vi "Inst_DS360.vi"(8 "error in":errorcluster, 10 "All Message Queues in":T1, 11 "AjustesPrevios in":refnum<class "AjustesPrevios.lvclass">) -> (0 "error out":errorcluster)   [LabVIEW 2019, in "AjustesPrevios.lvclass"]
uses:
  AjustesPrevios.lvclass
  QMH/Message Queue/All Message Queues.ctl
  QMH/Message Queue/Message Cluster.ctl
  AjustesPrevios.lvclass/AjustesPrevios.ctl
  <vilib>/Utility/error.llb/Error Cluster From Error Code.vi
  QMH/Message Queue/Enqueue Message (Single).vi
  <vilib>/ErrorRing/Error Ring.xnode
  QMH/Message Queue/Message Queue.lvlib
  Instrumento/DS360/DS360.lvclass
panel:
  out "All States":string[](array[string])
  out "Actual State":string
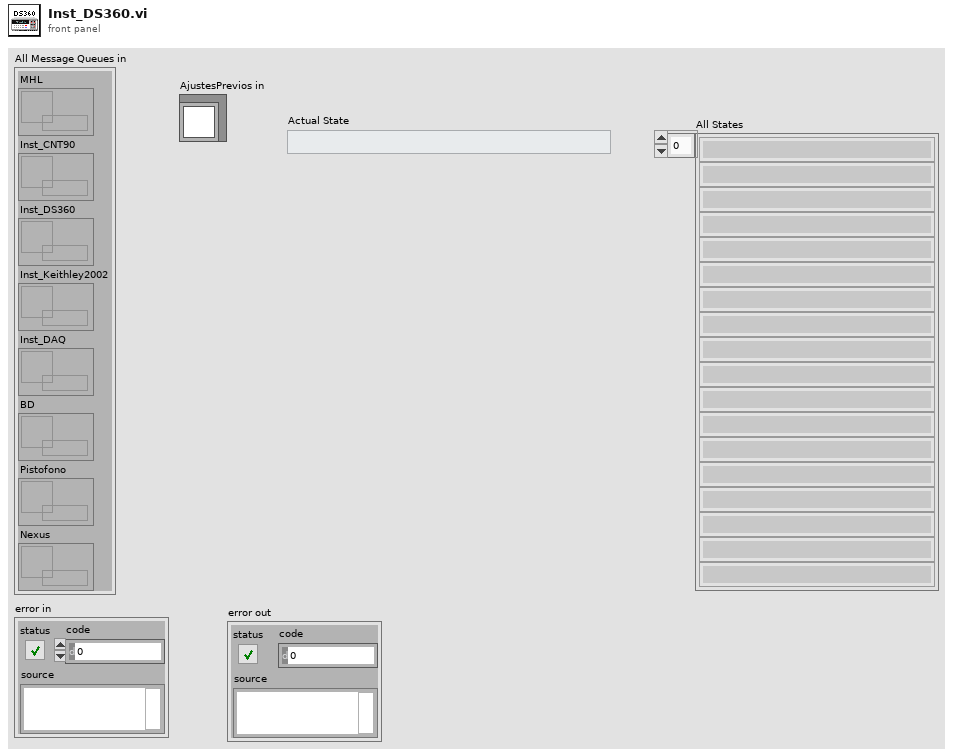
[diagram p1: front panel]
types:
  T1 = typedef "Message Queue.lvlib/All Message Queues.ctl" = cluster{"MHL":refnum<queue>, "Inst_CNT90":refnum<queue>, "Inst_DS360":refnum<queue>, "Inst_Keithley2002":refnum<queue>, "Inst_DAQ":refnum<queue>, "BD":refnum<queue>, "Pistofono":refnum<queue>, "Nexus":refnum<queue>}
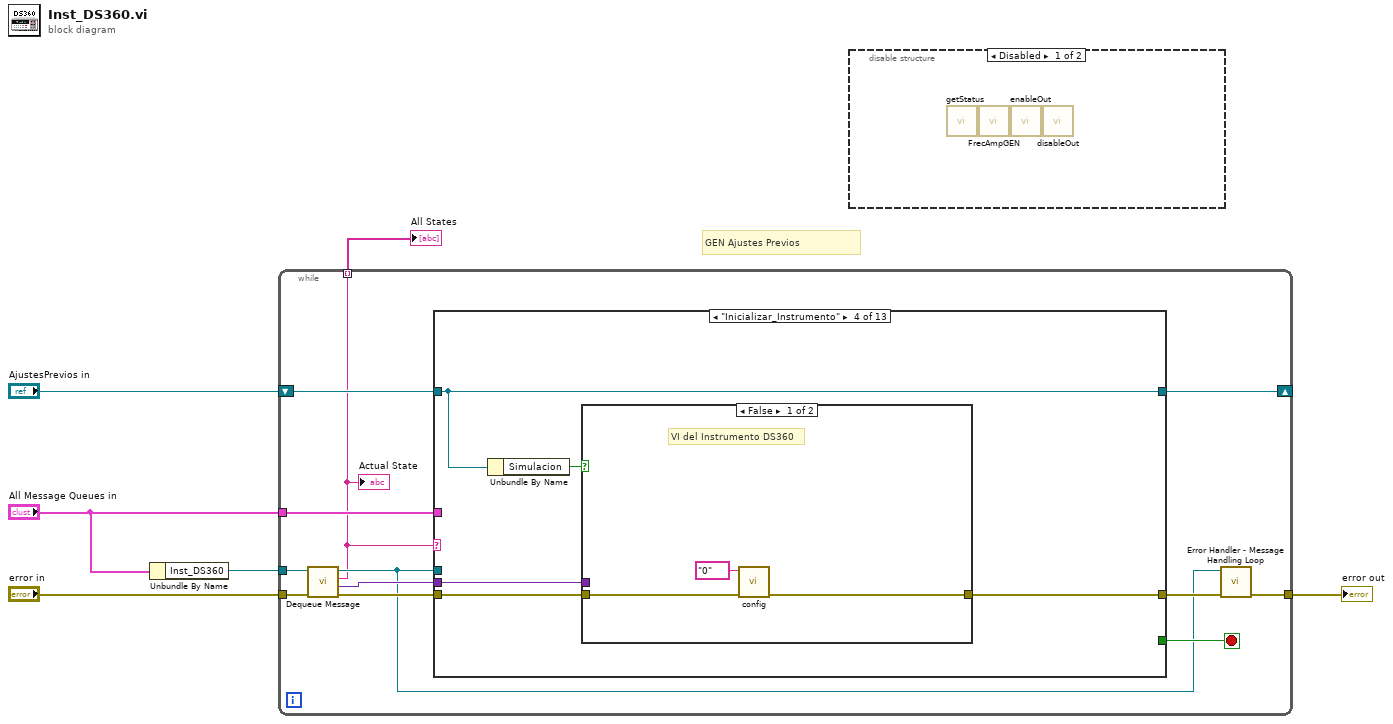
[diagram p0: block diagram]
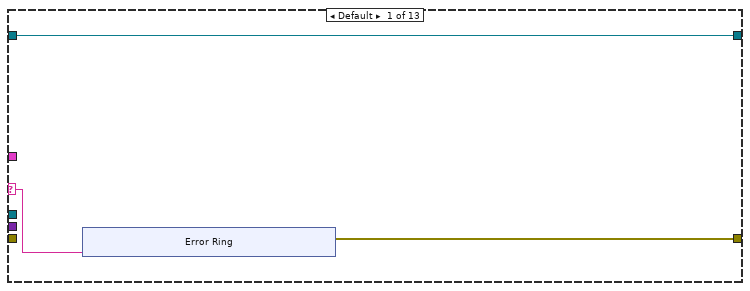
[diagram p3: hidden frame]
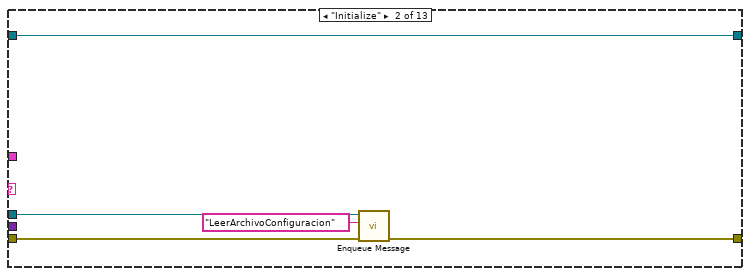
[diagram p4: hidden frame]
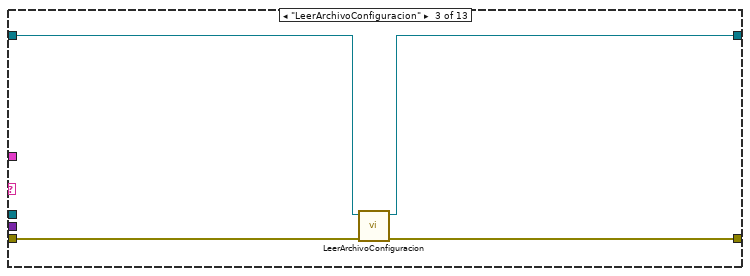
[diagram p5: hidden frame]
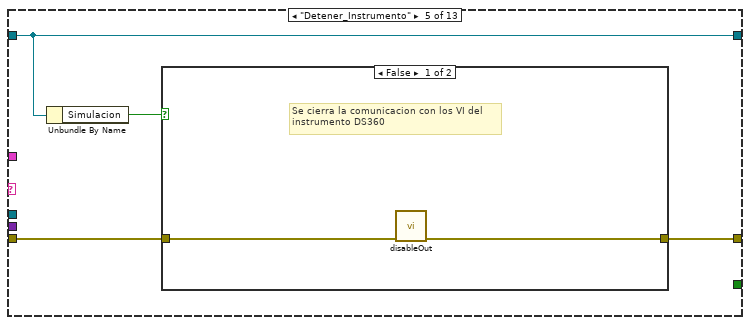
[diagram p7: hidden frame]
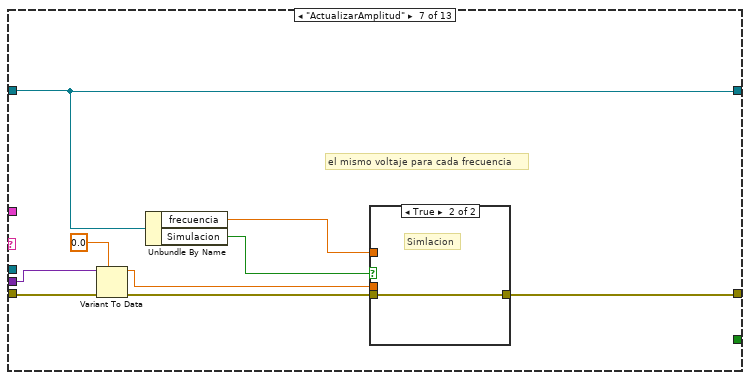
[diagram p10: hidden frame]
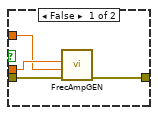
[diagram p11: hidden frame]
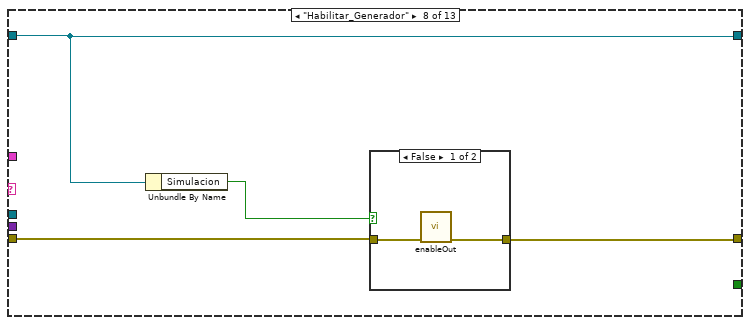
[diagram p12: hidden frame]
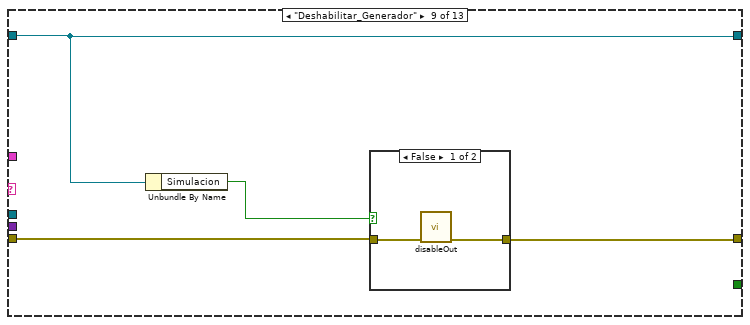
[diagram p14: hidden frame]
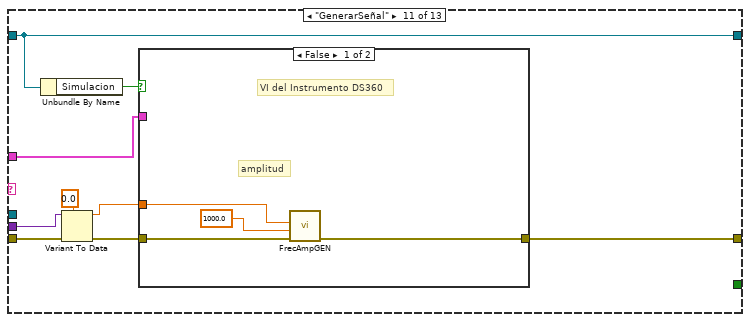
[diagram p17: hidden frame]
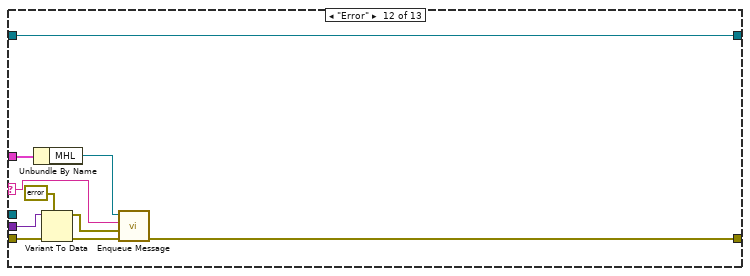
[diagram p19: hidden frame]
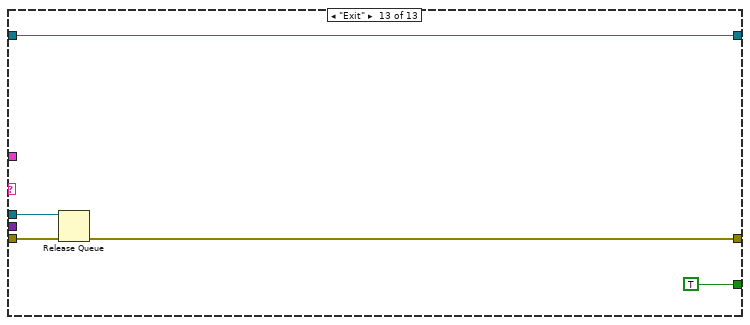
[diagram p20: hidden frame]
diagram:
  # "GEN Ajustes Previos"
  n1 = Unbundle By Name("All Message Queues in") -> ("Inst_DS360"=w4:refnum<queue>)
  n2 = while {
    tunnel: "error in" -> [w18]
    tunnel: w4 -> [w17]
    tunnel: "All Message Queues in" -> [w16]
    tunnel: [w9] -> w2
    shift-right: [w12] -> _
    shift-left: "AjustesPrevios in" -> [w15]
    tunnel: [w7] -> w1 mode=indexing
    stop <- w11 stop-if-true
    n3 = call "Dequeue Message.vi"("error in (no error)"=w18, "Message Queue"=w17) -> ("error out"=w13:errorcluster, "Message Data"=w14:variant, "Message"=w7:string, "dup Message Queue"=w8:refnum<queue>)  [unwired: 6 in]
    "Actual State" <- w7
    n4 = case shown="\"Inicializar_Instrumento\"" w7 {
      selector: w7 -> [w21 _ _ _ _ _ _ _ _ _ _ w102 _]
      tunnel: w16 -> [_ _ _ _ _ _ _ _ _ _ w92 w101 _]
      tunnel: w15 -> [w19 w33 w35 w40 w49 w55 w57 w70 w77 w84 w91 w109 w111]
      tunnel: w8 -> [_ w30 _ _ _ _ _ _ _ _ _ _ w113]
      tunnel: w14 -> [_ _ _ w39 _ _ w56 _ _ _ w88 w106 _]
      tunnel: w13 -> [_ w32 w37 w38 w47 w54 w59 w72 w79 w85 w93 w107 w114]
      tunnel: [w20 w31 w36 w42 w50 w54 w58 w71 w78 w85 w94 w104 w110] -> w10
      tunnel: [w19 w33 w34 w40 w49 w55 w57 w70 w77 w84 w91 w109 w111] -> w12
      tunnel: [_ _ _ _ _ _ _ _ _ _ _ _ TRUE] -> w11
      frame Default {
        n5 = xnode "Error Ring"("parameter 0"=w21) -> ("error out"=w20:errorcluster)
      }
      frame "Initialize" {
        n6 = call-poly "Enqueue Message.vi"("error in (no error)"=w32, "Message"="LeerArchivoConfiguracion", "Message Queue"=w30) -> ("error out"=w31:errorcluster)  [unwired: 7 in, 1 out]
      }
      frame "LeerArchivoConfiguracion" {
        n7 = call "LeerArchivoConfiguracion.vi"("error in"=w37, "AjustesPrevios in"=w35) -> ("error out"=w36:errorcluster, "AjustesPrevios out"=w34:refnum<class "AjustesPrevios.lvclass">)  [unwired: 8 in]
      }
      frame "Inicializar_Instrumento" {
        n8 = Unbundle By Name(w40) -> ("Simulacion"=w41:bool)
        n9 = case shown="False" w41 {
          tunnel: [w45 w46] -> w42
          tunnel: w38 -> [w44 w46]
          tunnel: w39 -> [_ _]
          frame False {
            # "VI del Instrumento DS360"
            n10 = call "config.vi"("error in (no error)"=w44, "Impedancia"="0") -> ("error out"=w45:errorcluster)  [unwired: 8 in, 1 out]
          }
          frame True {
            # "Simulacion"
          }
        }
      }
      frame "Detener_Instrumento" {
        n11 = Unbundle By Name(w49) -> ("Simulacion"=w48:bool)
        n12 = case shown="False" w48 {
          tunnel: [w52 w53] -> w50
          tunnel: w47 -> [w51 w53]
          frame False {
            # "Se cierra la comunicacion con los VI del\ninstrumento DS360"
            n13 = call "disableOut.vi"("error in (no error)"=w51) -> ("error out"=w52:errorcluster)  [unwired: 9 in, 1 out]
          }
          frame True {
            # "Simulacion"
          }
        }
      }
      frame "Leer_Instrumento" {
      }
      frame "ActualizarAmplitud" {
        # "el mismo voltaje para cada frecuencia"
        n14 = Variant To Data(error in=w59, type=0.0, Variant=w56) -> (data=w62:dbl, error out=w64:errorcluster)
        n15 = Unbundle By Name(w57) -> ("frecuencia"=w60:dbl, "Simulacion"=w61:bool)
        n16 = case shown="True" w61 {
          tunnel: [w68 w69] -> w58
          tunnel: w64 -> [w67 w69]
          tunnel: w62 -> [w66 _]
          tunnel: w60 -> [w65 _]
          frame False {
            n17 = call "FrecAmpGEN.vi"("error in (no error)"=w67, "Frec (Hz)"=w65, "Amplitud (Vrms)"=w66) -> ("error out"=w68:errorcluster)  [unwired: 7 in, 1 out]
          }
          frame True {
            # "Simlacion"
          }
        }
      }
      frame "Habilitar_Generador" {
        n18 = Unbundle By Name(w70) -> ("Simulacion"=w73:bool)
        n19 = case shown="False" w73 {
          tunnel: [w74 w76] -> w71
          tunnel: w72 -> [w75 w76]
          frame False {
            n20 = call "enableOut.vi"("error in (no error)"=w75) -> ("error out"=w74:errorcluster)  [unwired: 9 in, 1 out]
          }
          frame True {
            # "Simlacion"
          }
        }
      }
      frame "Deshabilitar_Generador" {
        n21 = Unbundle By Name(w77) -> ("Simulacion"=w80:bool)
        n22 = case shown="False" w80 {
          tunnel: [w81 w83] -> w78
          tunnel: w79 -> [w82 w83]
          frame False {
            n23 = call "disableOut.vi"("error in (no error)"=w82) -> ("error out"=w81:errorcluster)  [unwired: 9 in, 1 out]
          }
          frame True {
            # "Simlacion"
          }
        }
      }
      frame "No_Leer_Instrumento" {
      }
      frame "GenerarSeñal" {
        n24 = Unbundle By Name(w91) -> ("Simulacion"=w90:bool)
        n25 = Variant To Data(error in=w93, type=0.0 ("Frec (Hz)"), Variant=w88) -> (data=w86:dbl, error out=w89:errorcluster)
        n26 = case shown="False" w90 {
          tunnel: [w98 w99] -> w94
          tunnel: w89 -> [w97 w99]
          tunnel: w92 -> [_ _]
          tunnel: w86 -> [w95 _]
          frame False {
            # "amplitud"
            # "VI del Instrumento DS360"
            n27 = call "FrecAmpGEN.vi"("error in (no error)"=w97, "Frec (Hz)"=1000.0, "Amplitud (Vrms)"=w95) -> ("error out"=w98:errorcluster)  [unwired: 7 in, 1 out]
          }
          frame True {
            # "Simulacion"
          }
        }
      }
      frame "Error" {
        n28 = Unbundle By Name(w101) -> ("MHL"=w100:refnum<queue>)
        n29 = Variant To Data(error in=w107, type=errorcluster {"status"=FALSE, "code"=0, "source"=""} ("error constant"), Variant=w106) -> (data=w103:errorcluster, error out=w105:errorcluster)
        n30 = call-poly "Enqueue Message.vi"("error in (no error)"=w105, "Message Data"=w103, "Message"=w102, "Message Queue"=w100) -> ("error out"=w104:errorcluster)  [unwired: 6 in, 1 out]
      }
      frame "Exit" {
        n31 = Release Queue(queue=w113, error in (no error)=w114) -> (error out=w110:errorcluster)  [unwired: 1 in, 2 out]
      }
    }
    n32 = call "Error Handler - Message Handling Loop.vi"("error in (no error)"=w10, "Message Queue"=w8) -> ("dup error in"=w9:errorcluster)  [unwired: 8 in, 1 out]
  }
  "error out" <- w2
  "All States" <- w1
  n33 = disable-structure shown="Disabled" {
    frame Disabled {
      n34 = call "getStatus.vi"() -> ()  [unwired: 9 in, 3 out]
      n35 = call "FrecAmpGEN.vi"() -> ()  [unwired: 10 in, 2 out]
      n36 = call "enableOut.vi"() -> ()  [unwired: 10 in, 2 out]
      n37 = call "disableOut.vi"() -> ()  [unwired: 10 in, 2 out]
    }
    frame Enabled {
    }
  }
